vi "Test Simulator.vi"() -> ()   [LabVIEW 2017, in "Examples.lvlib"]
uses:
  Examples.lvlib
  <vilib>/Analysis/NI_AALBase.lvlib
panel:
  out "Test Signal":waveform(dbl)
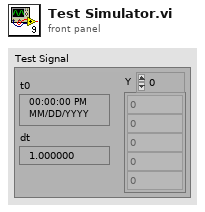
[diagram p1: front panel]
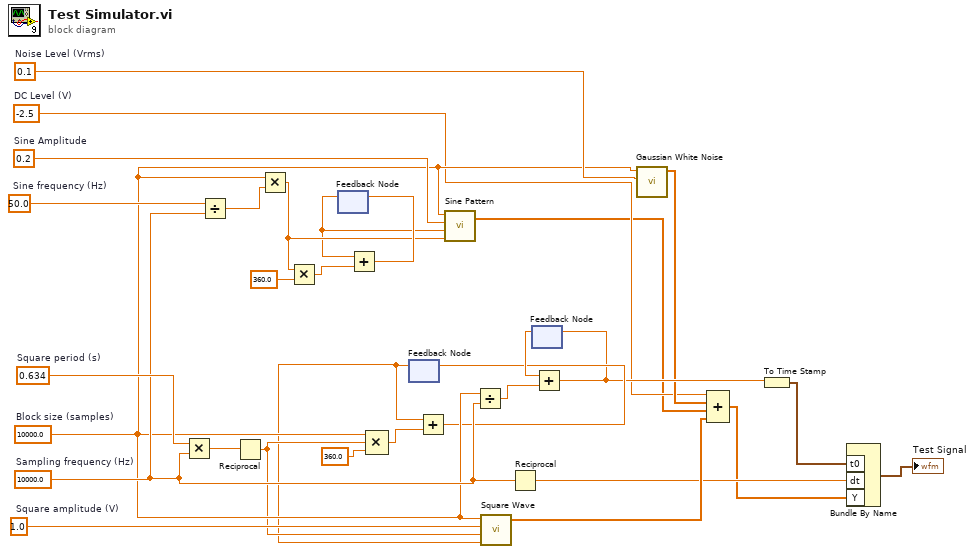
[diagram p0: block diagram]
diagram:
  w27 = 1.0  # Square amplitude (V)
  w16 = 10000.0  # Sampling frequency (Hz)
  w15 = 10000.0  # Block size (samples)
  w22 = 0.634  # Square period (s)
  w30 = 50.0  # Sine frequency (Hz)
  w21 = 0.2  # Sine Amplitude
  w9 = -2.5  # DC Level (V)
  w29 = 0.1  # Noise Level (Vrms)
  n1 = Multiply(x=w22, y=w16) -> (x*y=w23:dbl)
  n2 = Divide(x=w30, y=w16) -> (x/y=w28:dbl)
  n3 = Reciprocal(x=w23) -> (1/x=w8:dbl)
  n4 = Multiply(x=w15, y=w28) -> (x*y=w20:dbl)
  n5 = Multiply(x=w20, y=360.0) -> (x*y=w25:dbl)
  n6 = feedback #1() -> (w19:dbl)  [unwired: 1 in]
  n7 = Add(x=w19, y=w25) -> (x+y=w24:dbl)
  n8 = feedback-in #1(w24) -> ()
  n9 = Compound Arithmetic op=MULTIPLY(w15, w8, 360.0 ("value")) -> (w18:dbl)
  n10 = feedback #2() -> (w7:dbl)  [unwired: 1 in]
  n11 = Add(x=w7, y=w18) -> (x+y=w12:dbl)
  n12 = feedback-in #2(w12) -> ()
  n13 = call <vilib>:"Sine Pattern.vi"("cycles"=w20, "phase(degrees)"=w19, "amplitude"=w21, "samples"=w15) -> ("Sinusoidal Pattern"=w6:dbl[])  [unwired: 1 out]
  n14 = Divide(x=w15, y=w16) -> (x/y=w14:dbl)
  n15 = call <vilib>:"Square Wave.vi"("samples"=w15, "amplitude"=w27, "frequency"=w8, "phase in"=w7) -> ("square wave"=w5:dbl[])  [unwired: 2 in, 2 out]
  n16 = Reciprocal(x=w16) -> (1/x=w3:dbl)
  n17 = feedback #3() -> (w13:dbl)  [unwired: 1 in]
  n18 = Add(x=w13, y=w14) -> (x+y=w11:dbl)
  n19 = feedback-in #3(w11) -> ()
  n20 = call <vilib>:"Gaussian White Noise.vi"("standard deviation"=w29, "samples"=w15) -> ("Gaussian noise pattern"=w10:dbl[])  [unwired: 8 in, 1 out]
  n21 = Compound Arithmetic op=ADD(w9, w10, w6, w5) -> (w2:dbl[])
  n22 = To Time Stamp(1:w11) -> (0:w4:timestamp)
  n23 = Bundle By Name("t0"=w4, "dt"=w3, "Y"=w2) -> (→"Test Signal":waveform(dbl))  [unwired: 1 in]
